vi "getdonneespointage.vi"(1 "Fichier DB":string) -> (0 "Données pointage":string[][](table))   [LabVIEW 2024]
uses:
  <vilib>/drjdpowell/SQLite Library/SQLite.lvlib
  <vilib>/drjdpowell/SQLite Library/SQL Connection/Connection.lvclass
  <vilib>/drjdpowell/SQLite Library/SQL Connection/Execute SQL.vi
  <vilib>/drjdpowell/SQLite Library/SQL Connection/Open (string).vi
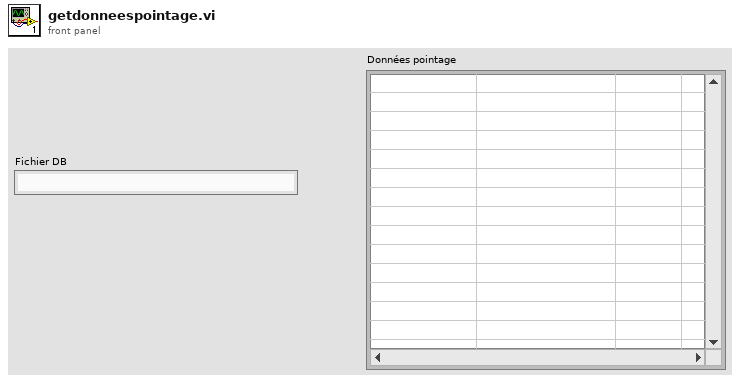
[diagram p1: front panel]
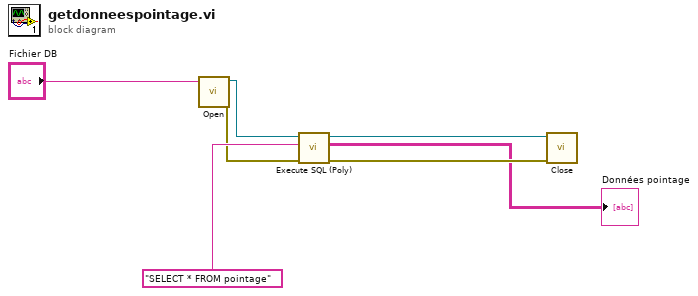
[diagram p0: block diagram]
diagram:
  n1 = call-poly <vilib>:"Open.vi"("db file"="Fichier DB") -> ("error out"=w2:errorcluster, "SQLite Connection"=w3:refnum<class "Connection.lvclass">)  [unwired: 9 in]
  n2 = call-poly <vilib>:"Execute SQL (Poly).vi"("error in (no error)"=w2, "SQL"="SELECT * FROM pointage", "SQLite Connection in"=w3) -> ("error out"=w6:errorcluster, "Result Set"=→"Données pointage":string[][], "SQLite Connection"=w7:refnum<class "Connection.lvclass">)  [unwired: 5 in, 1 out]
  n3 = call-dynamic "Close.vi"("error in (no error)"=w6, "SQLite Connection in"=w7) -> ()  [unwired: 9 in, 1 out]
